vi "ViperHawk Check Unit Software Version.vi"(8 "error in (no error)":errorcluster, 9 "GEA2 Event Registration":refnum<event-registration>, 10 "Board Index":i32, 11 "Input Data":T1={"Source"=37, "Destination"=33, "Command"=1, "Message"=""} {"Command" format="%02x"; "Destination" format="%02x"; "Source" format="%02x"}) -> (0 "error out":errorcluster, 1 "Event Registration Out":refnum<event-registration>, 3 "Software Version":T2)   [LabVIEW 2014]
uses:
  Utility/Save File/Public/Type Definitions/Save File Software Version.ctl
  Utility/LabVIEW GEA2 Toolkit v1.0.0.0/type defs/Data In.ctl
  Utility/LabVIEW GEA2 Toolkit v1.0.0.0/type defs/Data Out.ctl
  Utility/LabVIEW GEA2 Toolkit v1.0.0.0/library/GEA2_Toolkit.lvlib
  Utility/Save File/Save File.lvlib
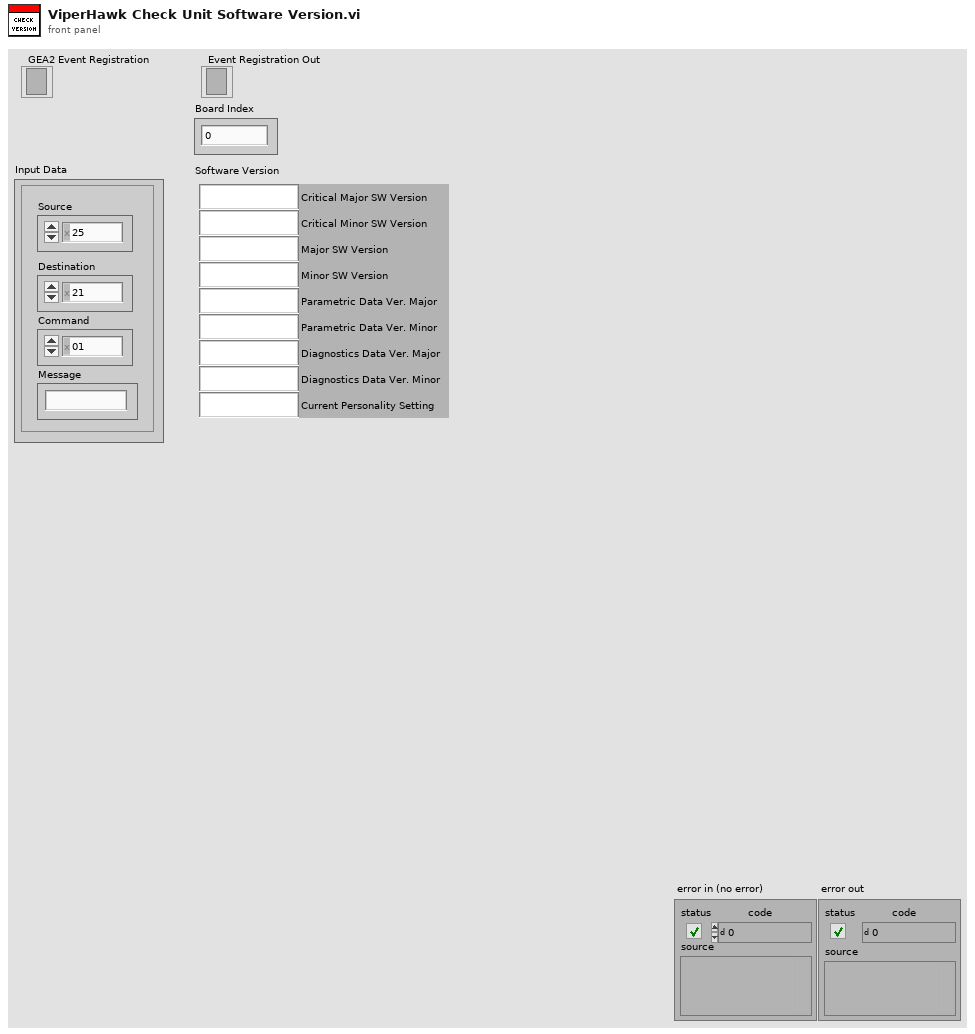
[diagram p1: front panel]
types:
  T1 = typedef "GEA2_Toolkit.lvlib/Data In.ctl" = cluster{"Source":u8, "Destination":u8, "Command":u8, "Message":string}
  T2 = typedef "Save File.lvlib/Save File Software Version.ctl" = cluster{"Critical Major SW Version":string, "Critical Minor SW Version":string, "Major SW Version":string, "Minor SW Version":string, "Parametric Data Ver. Major":string, "Parametric Data Ver. Minor":string, "Diagnostics Data Ver. Major":string, "Diagnostics Data Ver. Minor":string, "Current Personality Setting":string}
  T3 = typedef "GEA2_Toolkit.lvlib/Data Out.ctl" = cluster{"Source":u8, "Destination":u8, "Command":u8, "Length":u8, "CRC":u16, "Message":string}
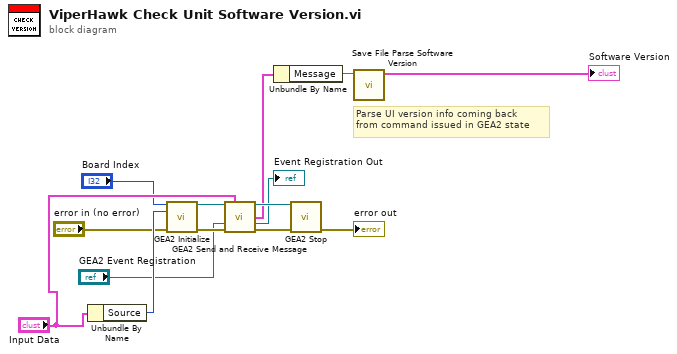
[diagram p0: block diagram]
diagram:
  # "Parse UI version info coming back\nfrom command issued in GEA2 state"
  n1 = Unbundle By Name("Input Data") -> ("Source"=w8:u8)
  n2 = call "GEA2 Initialize.vi"("Board Index"="Board Index", "Source Address"=w8, "error in"="error in (no error)") -> ("GEA2 Reference Out"=w12:refnum<k24>, "error out"=w9:errorcluster)  [unwired: 10 in, 1 out]
  n3 = call "GEA2 Send and Receive Message.vi"("GEA2 Reference In"=w12, "Input Data"="Input Data", "GEA2 Event Registration"="GEA2 Event Registration", "Error In"=w9) -> ("GEA2 Reference Out"=w11:refnum<k24>, "Converted Data Out"=w7:T3, "Event Registration Out"=→"Event Registration Out":refnum<event-registration>, "Error Out"=w10:errorcluster)  [unwired: 7 in, 1 out]
  n4 = Unbundle By Name(w7) -> ("Message"=w13:string)
  n5 = call "GEA2 Stop.vi"("GEA2 Reference Out"=w11, "Error In"=w10) -> ("Error Out"=→"error out":errorcluster)  [unwired: 13 in]
  n6 = call "Save File Parse Software Version.vi"("Message"=w13) -> ("UI Version"=→"Software Version":T2)  [unwired: 10 in]
